vi "TagHTMLContent.vi"(1 "Escape Contents":bool, 2 "Tag":string, 3 "Element Contents":string) -> (0 "Tagged Contents":string)   [LabVIEW 2017, in "ArgosLib.lvlib"]
uses:
  ArgosLib.lvlib
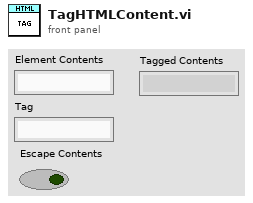
[diagram p1: front panel]
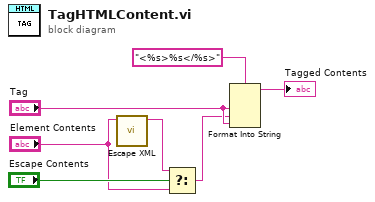
[diagram p0: block diagram]
diagram:
  n1 = call <vilib>:"Escape XML.vi"("XML String In"="Element Contents") -> ("XML String Out"=w5:string)  [unwired: 9 in, 1 out]
  n2 = Select(t=w5, s="Escape Contents", f="Element Contents") -> (s? t:f=w3:string)
  n3 = Format Into String(format string="<%s>%s</%s>", "Tag", w3, "Tag") -> (resulting string=→"Tagged Contents":string)  [unwired: 2 in, 1 out]
